vi "runCamController.vi"(8 "error in (no error)":errorcluster, 11 "CameraManager in":refnum<class "CameraManager.lvclass">) -> (0 "error out":errorcluster, 3 "CameraManager out":refnum<class "CameraManager.lvclass">)   [LabVIEW 2011, in "iManagement.lvlib" / "CameraManager.lvclass"]
uses:
  CameraManager.lvclass
  CameraManager.lvclass/CameraManager.ctl
  Hal/Channels/Camera/CameraController.lvclass
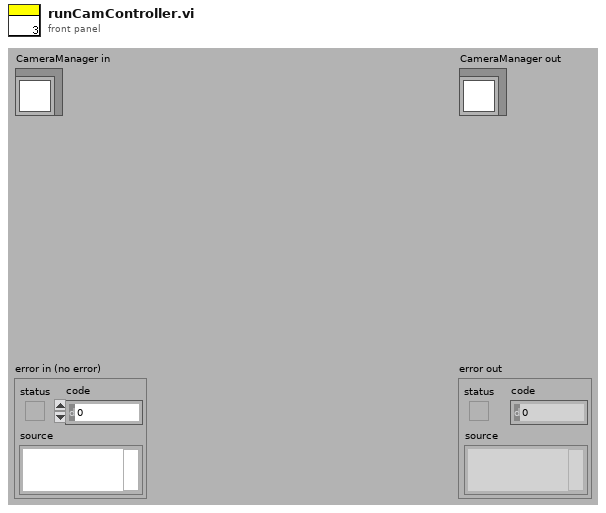
[diagram p1: front panel]
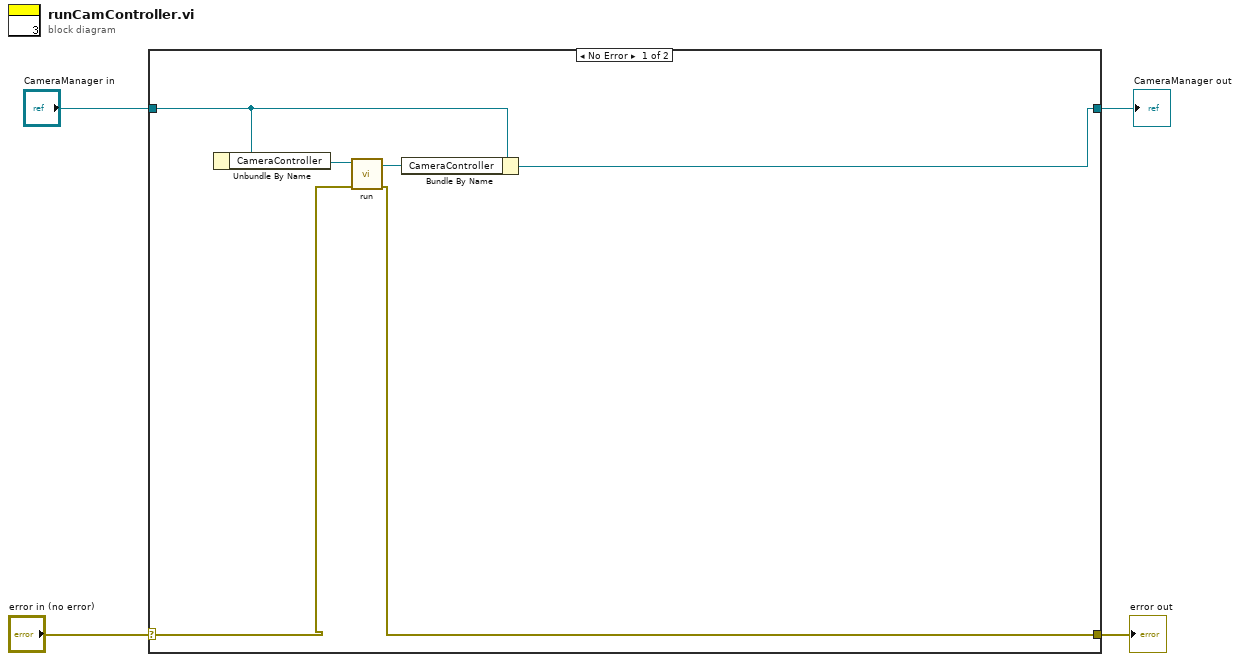
[diagram p0: block diagram]
diagram:
  n1 = case shown="No Error" "error in (no error)" {
    selector: "error in (no error)" -> [w6 w12]
    tunnel: [w5 w12] -> w3
    tunnel: [w7 w11] -> w1
    tunnel: "CameraManager in" -> [w8 w11]
    frame No Error {
      n2 = Unbundle By Name(w8) -> ("CameraController"=w10:refnum<class "CameraController.lvclass">)
      n3 = call-dynamic "run.vi"("error in (no error)"=w6, "CameraController in"=w10) -> ("error out"=w5:errorcluster, "CameraController out"=w9:refnum<class "CameraController.lvclass">)  [unwired: 7 in, 1 out]
      n4 = Bundle By Name(cluster=w8, "CameraController"=w9) -> (w7:refnum<class "CameraManager.lvclass">)
    }
    frame Error {
    }
  }
  "error out" <- w3
  "CameraManager out" <- w1
